vi "Read Label.vi"(8 "error in (no error)":errorcluster, 11 "Message":refnum<class "VarMessage.lvclass">) -> (0 "error out":errorcluster, 2 "Label":string caption="Label (or Data Name)", 3 "Message":refnum<class "VarMessage.lvclass">)   [LabVIEW 2011, in "Messenging.lvlib" / "VarMessage.lvclass"]
uses:
  VarMessage.lvclass
  TextVarientMessage/MSG.lvclass
panel:
  # "Uses name of data in Varient if Label is empty"
  # "Aug 26, 2011 (LabVIEW 8.6.1) BUG invloving LabVIEW keeping the data name\nof a previous variant when type-casting into the \"Write VarMessage\" VI\n\nThus this method is not relyable.   -- JDP"
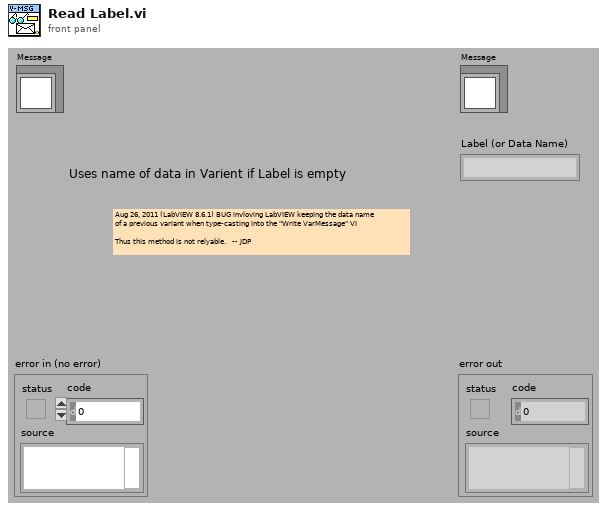
[diagram p1: front panel]
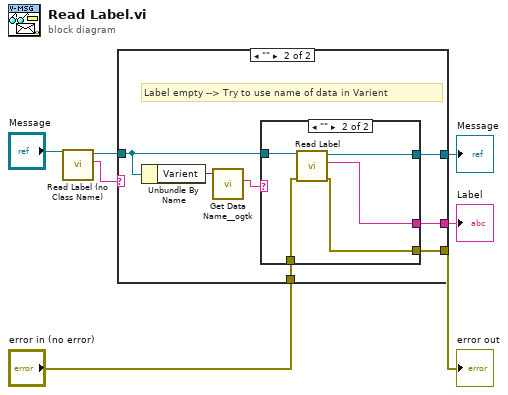
[diagram p0: block diagram]
diagram:
  n1 = call "Read Label (no Class Name).vi"("MSG.lvclass in"="Message") -> ("Label"=w6:string, "MSG.lvclass out"=w5:refnum<class "VarMessage.lvclass">)  [unwired: 9 out]
  n2 = case shown="\"\"" w6 {
    selector: w6 -> [w9 _]
    tunnel: w5 -> [w10 w15]
    tunnel: [w9 w14] -> w4
    tunnel: [w10 w13] -> w3
    tunnel: [w8 w12] -> w2
    tunnel: "error in (no error)" -> [w8 w11]
    frame "False", Default {
    }
    frame "" {
      # "Label empty --> Try to use name of data in Varient"
      n3 = Unbundle By Name(w15) -> ("Varient"=w17:variant)
      n4 = call <userlib>:"Get Data Name__ogtk.vi"("Data"=w17) -> ("Data Name"=w16:string)  [unwired: 1 in, 9 out]
      n5 = case shown="\"\"" w16 {
        selector: w16 -> [w19 _]
        tunnel: w15 -> [w20 w25]
        tunnel: [w19 w24] -> w14
        tunnel: [w20 w23] -> w13
        tunnel: [w18 w21] -> w12
        tunnel: w11 -> [w18 w22]
        frame Default {
        }
        frame "" {
          n6 = call-parent "Read Label.vi"("error in (no error)"=w22, "Message"=w25) -> ("error out"=w21:errorcluster, "Label"=w24:string, "Message"=w23:refnum<class "VarMessage.lvclass">)  [unwired: 7 out]
        }
      }
    }
  }
  "error out" <- w2
  "Message" <- w3
  "Label" <- w4
